vi "Image_capture_V1.2.vi"() -> ()   [LabVIEW 2024]
panel:
  in  "Acquisition Control::Exposure Time":dbl=15004.0 min=100.0 max=29999995.0 step=200.0 format="%#_5g"
  in  "Analog Control::Gamma":dbl=0.800048828125 min=0.05 max=4.0 step=0.05 format="%#_4g"
  in  "Analog Control::Black Level 2":dbl caption="Analog Control::Black Level" min=-10.0 max=10.000002384185791 step=0.5 format="%#_4g"
  in  "Analog Control::Gain":dbl min=0.0 max=27.045663671679687 step=0.5 format="%#_3g"
  in  "Stop (F) 2":bool caption="Stop (F)"
  out "Image Out 2":T1(plugin-control)
  in  "File Path":path
  in  "Image Quality":u32=750 max=1000 step=10
  in  "Take image":bool
  out "error out 2":errorcluster
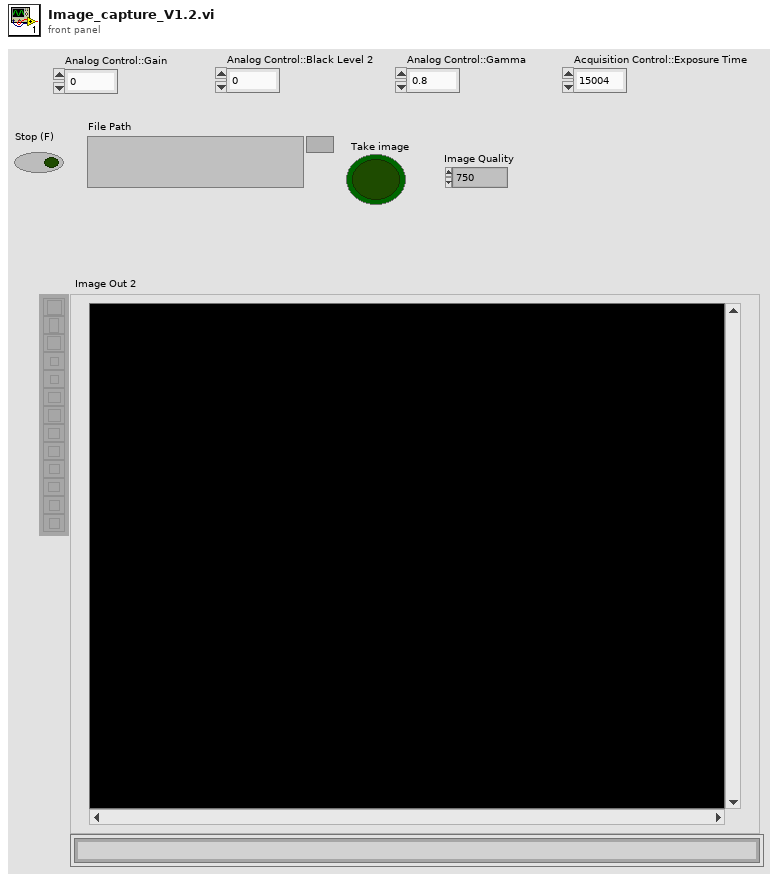
[diagram p1: front panel]
types:
  T1 = typedef "IMAQ Image.ctl" = refnum<image>
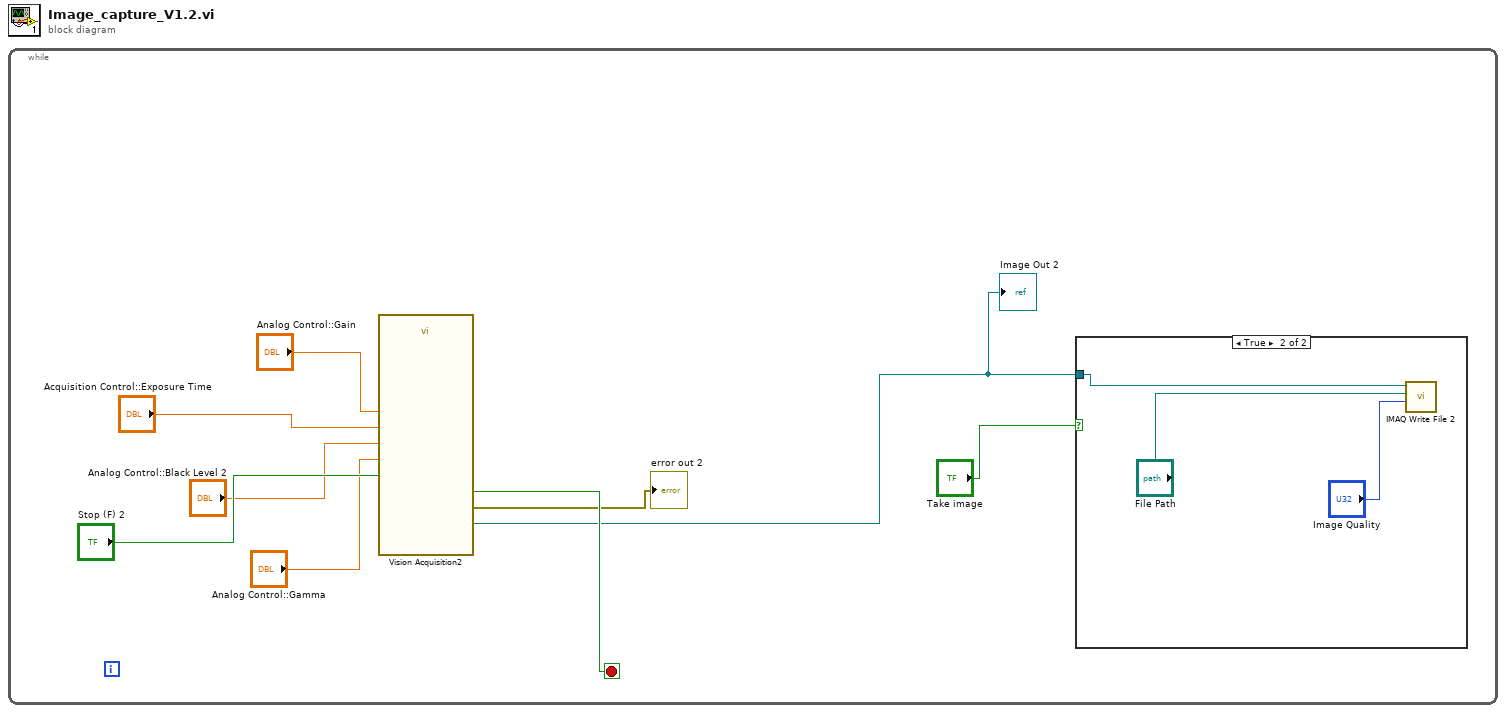
[diagram p0: block diagram]
diagram:
  n1 = while {
    stop <- w4 stop-if-true
    n2 = call "Vision Acquisition2"("Analog Control::Gain"="Analog Control::Gain", "Analog Control::Black Level"="Analog Control::Black Level 2", "Analog Control::Gamma"="Analog Control::Gamma", "Acquisition Control::Exposure Time"="Acquisition Control::Exposure Time", "Stop (F)"="Stop (F) 2") -> ("Image Out"=w2:T1, "Stopped"=w4:bool, "error out"=→"error out 2":errorcluster)  [unwired: 20 in]
    "Image Out 2" <- w2
    n3 = case shown="True" "Take image" {
      tunnel: w2 -> [_ w10]
      frame False {
      }
      frame True {
        n4 = call-poly "IMAQ Write File 2"("Image Quality"="Image Quality", "File Path"="File Path", "Image"=w10) -> ()  [unwired: 7 in, 2 out]
      }
    }
  }
